vi "Regression.vi"() -> ()   [LabVIEW 2019]
uses:
  <vilib>/Analysis/6fits.llb/1D B-Spline Fit.vi
  <vilib>/Analysis/NI_AALPro.lvlib
panel:
  in  "DataSet":bool
  out "B-Spline fit error":i32
  out "B-Spline Fit":T1(graph)
  out "Polynomial FIt Error":i32
  out "Polynomial Fit":T1(graph)
  out "Linear Error":i32
  out "Linear Fit":T1(graph)
  out "Cubic Spline Error":i32
  in  "stop":bool
  out "Cubic Spline Fit":T1(graph)
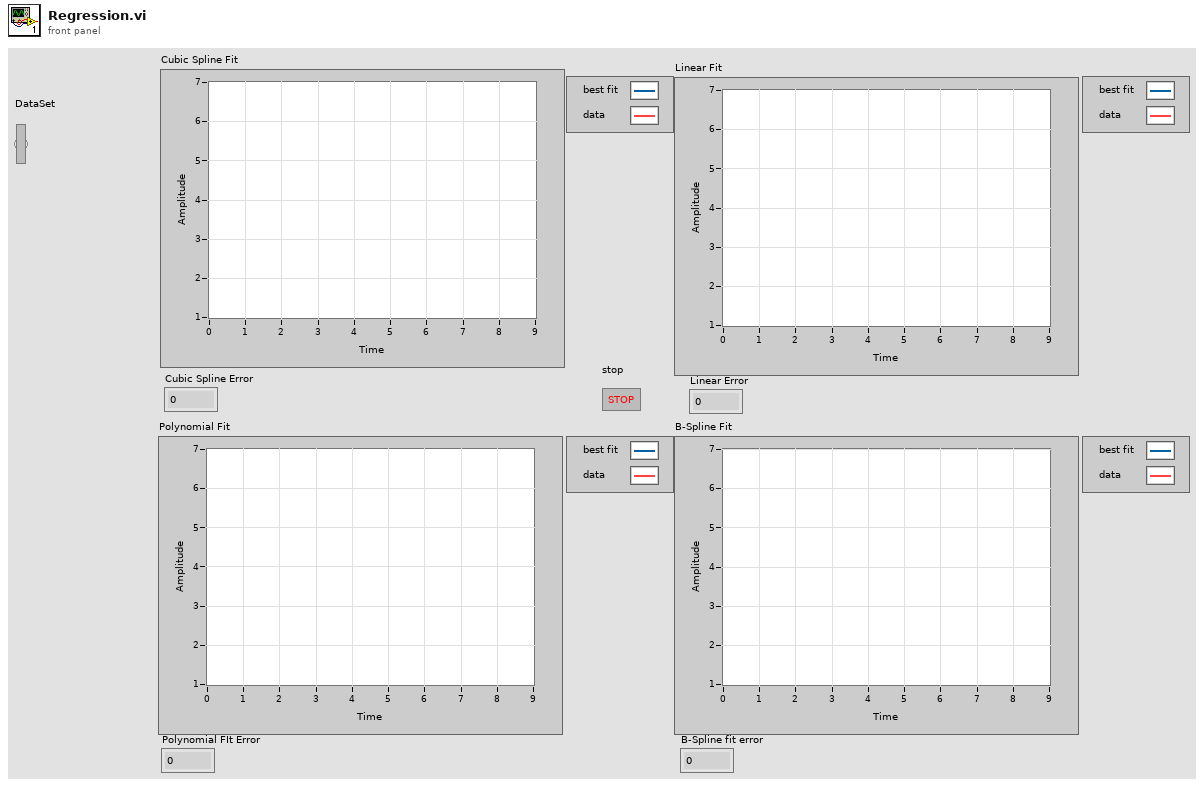
[diagram p1: front panel]
types:
  T1 = cluster{"Ramp Pattern":dbl[], "Best Linear Fit":dbl[]}[]
  T2 = cluster{"Sinc Pattern":dbl[], "Best Polynomial Fit":dbl[]}
  T3 = cluster{"Sinc Pattern":dbl[], "Best Cubic Spline Fit":dbl[]}
  T4 = cluster{"Sinc Pattern":dbl[], "Best Linear Fit":dbl[]}
  T5 = cluster{"Sinc Pattern":dbl[], "Best BSpline Fit Y":dbl[]}
  T6 = cluster{"Sinc Pattern":dbl[], "Sinc Pattern":dbl[]}
  T7 = cluster{"Sinc Pattern":dbl[], "Sinc Pattern":dbl[]}[]
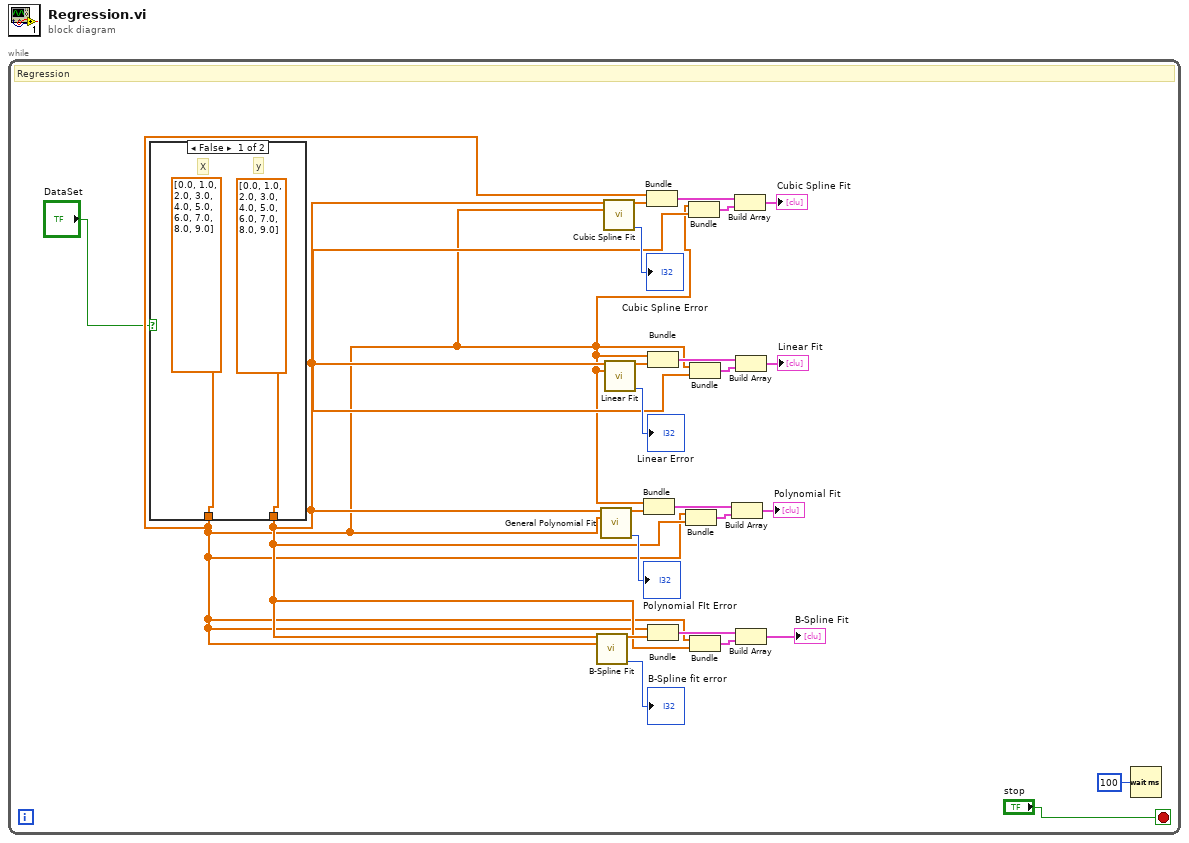
[diagram p0: block diagram]
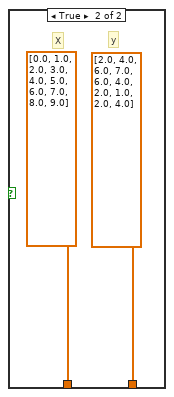
[diagram p2: hidden frame]
diagram:
  n1 = while {
    stop <- "stop" stop-if-true
    # "Regression"
    n2 = case shown="False" "DataSet" {
      tunnel: [dbl[] [0.0, 1.0, 2.0, 3.0, 4.0, 5.0, 6.0, 7.0, 8.0, 9.0] ("Sinc Pattern") dbl[] [2.0, 4.0, 6.0, 7.0, 6.0, 4.0, 2.0, 1.0, 2.0, 4.0] ("Sinc Pattern")] -> w3
      tunnel: [dbl[] [0.0, 1.0, 2.0, 3.0, 4.0, 5.0, 6.0, 7.0, 8.0, 9.0] ("Sinc Pattern") dbl[] [0.0, 1.0, 2.0, 3.0, 4.0, 5.0, 6.0, 7.0, 8.0, 9.0] ("Sinc Pattern")] -> w2
      frame False {
        # "y"
        # "X"
      }
      frame True {
        # "y"
        # "X"
      }
    }
    n3 = call-poly <vilib>:"B-Spline Fit.vi"("Y"=w3, "X"=w2) -> ("Best BSpline Fit Y"=w4:dbl[], "error"=→"B-Spline fit error":i32)  [unwired: 10 in, 2 out]
    n4 = call <vilib>:"General Polynomial Fit.vi"("Y"=w3, "X"=w2) -> ("Best Polynomial Fit"=w10:dbl[], "error"=→"Polynomial FIt Error":i32)  [unwired: 10 in, 2 out]
    n5 = call <vilib>:"Cubic Spline Fit.vi"("Y"=w3, "X"=w2) -> ("Best Cubic Spline Fit"=w22:dbl[], "error"=→"Cubic Spline Error":i32)  [unwired: 12 in]
    n6 = call <vilib>:"Linear Fit.vi"("Y"=w3, "X"=w2) -> ("Best Linear Fit"=w15:dbl[], "error"=→"Linear Error":i32)  [unwired: 9 in, 3 out]
    n7 = Bundle("Sinc Pattern"=w2, "Best Polynomial Fit"=w10) -> (w13:T2)  [unwired: 1 in]
    n8 = Bundle("Sinc Pattern"=w2, "Best Cubic Spline Fit"=w22) -> (w24:T3)  [unwired: 1 in]
    n9 = Bundle("Sinc Pattern"=w2, "Best Linear Fit"=w15) -> (w18:T4)  [unwired: 1 in]
    n10 = Bundle("Sinc Pattern"=w2, "Best BSpline Fit Y"=w4) -> (w8:T5)  [unwired: 1 in]
    n11 = Bundle("Sinc Pattern"=w2, "Sinc Pattern"=w3) -> (w12:T6)  [unwired: 1 in]
    n12 = Bundle("Sinc Pattern"=w2, "Sinc Pattern"=w3) -> (w21:T6)  [unwired: 1 in]
    n13 = Bundle("Sinc Pattern"=w2, "Sinc Pattern"=w3) -> (w17:T6)  [unwired: 1 in]
    n14 = Bundle("Sinc Pattern"=w2, "Sinc Pattern"=w3) -> (w7:T6)  [unwired: 1 in]
    n15 = Build Array(w13, w12) -> (→"Polynomial Fit":T7)
    n16 = Build Array(w24, w21) -> (→"Cubic Spline Fit":T7)
    n17 = Build Array(w18, w17) -> (→"Linear Fit":T7)
    n18 = Build Array(w8, w7) -> (→"B-Spline Fit":T7)
    n19 = Wait (ms)(milliseconds to wait=u32 100) -> ()  [unwired: 1 out]
  }
